vi "test Verify Scripting Code.LUnit.vi"(8 "error in":errorcluster, 11 "Test Case In":refnum<class "LUnit Extensions Tests.lvclass">) -> (0 "error out":errorcluster, 3 "Test Case Out":refnum<class "LUnit Extensions Tests.lvclass">)   [LabVIEW 2026, in "LUnit Extensions Tests.lvclass"]
uses:
  LUnit Extensions Tests.lvclass
  usr/local/natinst/LabVIEW-2026-64/vi.lib/Astemes/LUnit/Test Case.lvclass
  Source/Extensions/LUnit.Extension/LUnit.Extension.lvlib
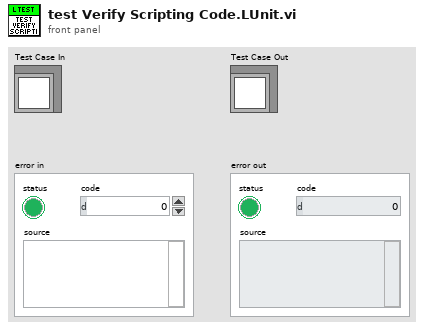
[diagram p1: front panel]
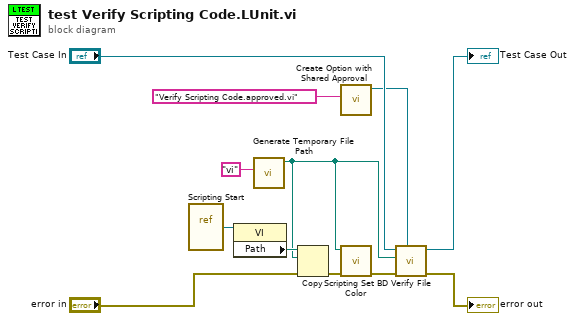
[diagram p0: block diagram]
diagram:
  n1 = vi-ref "Scripting Start.vi"() -> (w6:refnum<vi>)
  n2 = property on="Property Node" class="VI"(reference=w6) -> ("Path"=w4:path)  [unwired: 1 in, 2 out]
  n3 = call <vilib>:"Generate Temporary File Path.vi"("Temporary File Extension (tmp)"="vi") -> ("Unique Temporary File Path"=w3:path)  [unwired: 9 in, 1 out]
  n4 = Copy(8:"error in", 10:w3, 11:w4) -> (0:w9:errorcluster)  [unwired: 2 in, 2 out]
  n5 = call "Create Option with Shared Approval.vi"("Filename"="Verify Scripting Code.approved.vi") -> ("Options outs"=w1:refnum<class "Options.lvclass">)  [unwired: 10 in]
  n6 = call "Scripting Set BD Color.vi"("error in"=w9, "Path"=w3) -> ("error out"=w10:errorcluster)  [unwired: 9 in]
  n7 = call "Verify File.vi"("Options"=w1, "error in"=w10, "path to file"=w3, "LUnit Test Case In"="Test Case In") -> ("error out"=→"error out":errorcluster, "LUnit Test Case Out"=→"Test Case Out":refnum<class "LUnit Extensions Tests.lvclass">)  [unwired: 6 in]
